vi "Release.vi"(8 "error in (no error)":errorcluster, 11 "Data Buffer in":refnum<class "Data Buffer DBL.lvclass">) -> (0 "error out":errorcluster)   [LabVIEW 2020, in "VolatusData.lvlib" / "Data Buffer DBL.lvclass"]
uses:
  Data Buffer DBL.lvclass
  Data Buffer DBL.lvclass/Data Buffer DBL.ctl
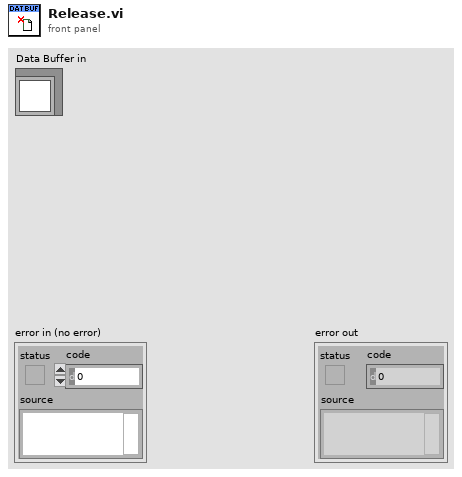
[diagram p1: front panel]
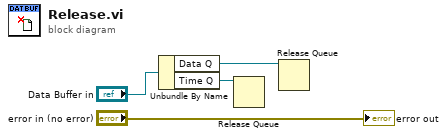
[diagram p0: block diagram]
diagram:
  n1 = Unbundle By Name("Data Buffer in") -> ("Data Q"=w1:refnum<queue>, "Time Q"=w2:refnum<queue>)
  n2 = Release Queue(queue=w2) -> ()  [unwired: 2 in, 3 out]
  n3 = Release Queue(queue=w1) -> ()  [unwired: 2 in, 3 out]
  "error out" <- "error in (no error)"
